vi "Map.vi"(7 "Action":enum8{"noop", "get", "set", "pop"}(ring), 9 "Is Registered in":bool, 10 "User Event in":refnum<user-event>, 11 "User Event Name":string) -> (0 "Found?":bool, 1 "Is Registered out":bool, 2 "User Event out":refnum<user-event>, 3 "User Event Map":T1(c390))   [LabVIEW 2021, in "UserEvent.lvlib"]
uses:
  UserEvent.lvlib
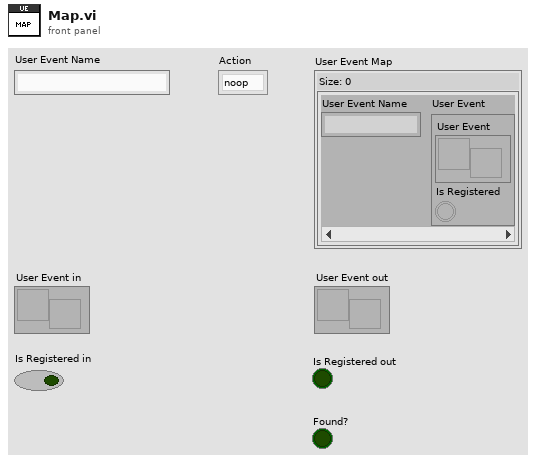
[diagram p1: front panel]
types:
  T1 = map{string, cluster{"User Event":refnum<user-event>, "Is Registered":bool}}
  T2 = cluster{"User Event in":refnum<user-event>, "Is Registered in":bool}
  T3 = cluster{"User Event":refnum<user-event>, "Ready":bool}
  T4 = cluster{"User Event":refnum<user-event>, "Is Registered":bool}
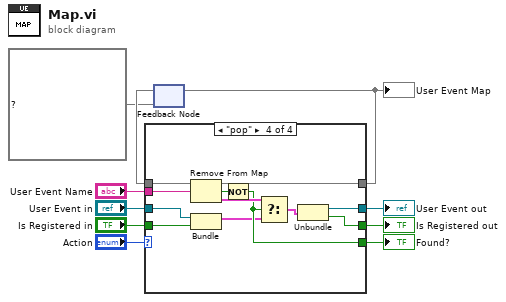
[diagram p0: block diagram]
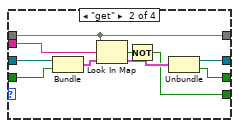
[diagram p3: hidden frame]
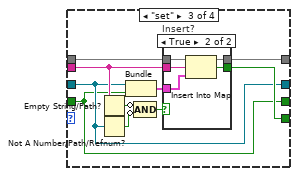
[diagram p4: hidden frame]
diagram:
  n1 = feedback #1(T1 {} ("User Event Map")) -> (w8:T1)
  n2 = case shown="\"pop\"" "Action" {
    tunnel: [w12 w15 w26 w41] -> w10
    tunnel: "User Event Name" -> [_ w21 w33 w49]
    tunnel: w8 -> [w13 w23 w32 w51]
    tunnel: [w13 w23 w31 w50] -> w7
    tunnel: [_ w18 w27 w44] -> w6
    tunnel: "User Event in" -> [w12 w22 w26 w47]
    tunnel: "Is Registered in" -> [w11 w16 w25 w42]
    tunnel: [w11 w14 w25 w40] -> w1
    frame "noop" {
    }
    frame "get" {
      n3 = Bundle("User Event in"=w22, "Is Registered in"=w16) -> (w17:T2)  [unwired: 1 in]
      n4 = Look In Map(map=w23, key=w21, default value=w17) -> (key not found?=w19:bool, value=w20:T3)
      n5 = Not(x=w19) -> (.not. x?=w18:bool)
      n6 = Unbundle(w20) -> ("User Event"=w15:refnum<user-event>, "Ready"=w14:bool)
    }
    frame "set" {
      n7 = Empty String/Path?(string/path=w33) -> (empty?=w30:bool)
      n8 = Not A Number/Path/Refnum?(number/path/refnum=w26) -> (NaN/Path/Refnum?=w28:bool)
      n9 = Bundle("User Event in"=w26, "Is Registered in"=w25) -> (w24:T2)  [unwired: 1 in]
      n10 = Compound Arithmetic op=AND(invert w30, invert w28) -> (w29:bool)
      n11 = case "Insert?" shown="True" w29 {
        tunnel: w32 -> [w34 w39]
        tunnel: w24 -> [_ w38]
        tunnel: w33 -> [_ w37]
        tunnel: [w34 w36] -> w31
        tunnel: [_ w35] -> w27
        frame False {
        }
        frame True {
          n12 = Insert Into Map(map in=w39, key=w37, value=w38) -> (map out=w36:T1, key already included?=w35:bool)  [unwired: 1 out]
        }
      }
    }
    frame "pop" {
      n13 = Remove From Map(10:w49, 11:w51) -> (1:w46:T4, 2:w48:bool, 3:w50:T1)
      n14 = Bundle("User Event in"=w47, "Is Registered in"=w42) -> (w43:T2)  [unwired: 1 in]
      n15 = Not(x=w48) -> (.not. x?=w44:bool)
      n16 = Select(t=w46, s=w44, f=w43) -> (s? t:f=w45:T2)
      n17 = Unbundle(w45) -> ("User Event in"=w41:refnum<user-event>, "Is Registered in"=w40:bool)
    }
  }
  "User Event out" <- w10
  "Found?" <- w6
  "User Event Map" <- w7
  "Is Registered out" <- w1
  n18 = feedback-in #1(w7) -> ()
